vi "Set Trig Type.vi"(7 "Requested state of Trig (off: Update)":bool, 11 "machine":T1 {"TimeStamp" format="%.2f"}) -> (0 "error out":errorcluster, 3 "Reply data":string)   [LabVIEW 2020]
uses:
  DataSocketCluster external.ctl
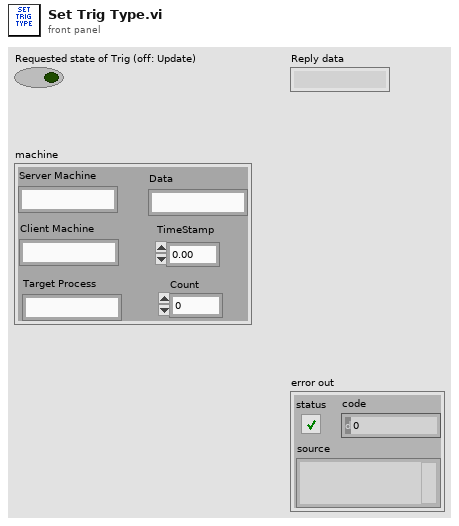
[diagram p1: front panel]
types:
  T1 = typedef "DataSocketCluster external.ctl" = cluster{"Server Machine":string, "Client Machine":string, "Data":string, "TimeStamp":dbl, "Count":i32, "Target Process":string}
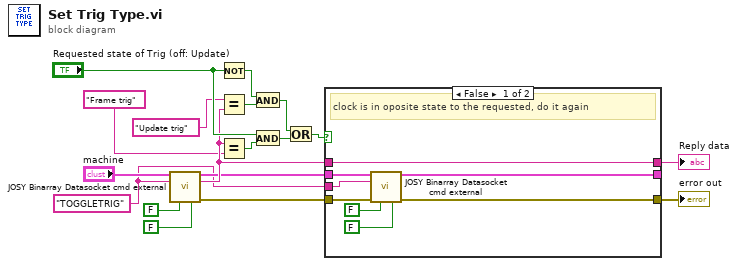
[diagram p0: block diagram]
diagram:
  w3 = "TOGGLETRIG" ("Command")
  n1 = call "JOSY Binarray Datasocket cmd external.vi"("DataSocketCluster In"="machine", "Command"=w3, "Command has variable"=FALSE, "String"=FALSE) -> ("DataSocketCluster Out"=w9:T1, "Reply data"=w13:string, "error out"=w17:errorcluster)  [unwired: 8 in, 1 out]
  n2 = Not(x="Requested state of Trig (off: Update)") -> (.not. x?=w14:bool)
  n3 = Equal?(x="Update trig" ("Reply data"), y=w13) -> (x = y?=w11:bool)
  n4 = Equal?(x=w13, y="Frame trig" ("Reply data")) -> (x = y?=w7:bool)
  n5 = And(x=w14, y=w11) -> (x .and. y?=w12:bool)
  n6 = And(x="Requested state of Trig (off: Update)", y=w7) -> (x .and. y?=w10:bool)
  n7 = Or(x=w12, y=w10) -> (x .or. y?=w16:bool)
  n8 = case shown="False" w16 {
    tunnel: [w20 w29] -> w8
    tunnel: w13 -> [w20 w29]
    tunnel: w9 -> [w24 w28]
    tunnel: [w23 w28] -> _
    tunnel: w17 -> [w22 w27]
    tunnel: [w21 w27] -> w18
    tunnel: w3 -> [w19 _]
    frame False {
      # "clock is in oposite state to the requested, do it again"
      n9 = call "JOSY Binarray Datasocket cmd external.vi"("DataSocketCluster In"=w24, "Command"=w19, "error in (no error)"=w22, "Command has variable"=FALSE, "String"=FALSE) -> ("DataSocketCluster Out"=w23:T1, "error out"=w21:errorcluster)  [unwired: 7 in, 2 out]
    }
    frame True {
      # "clock is as user wanted, nothing to do"
    }
  }
  "error out" <- w18
  "Reply data" <- w8
